vi "Logging Tree Contains.vi"(2 "Name":string, 3 "TreeRef":refnum<vi>) -> (0 "Contained":bool, 1 "TreeRef":refnum<vi>)   [LabVIEW 2012]
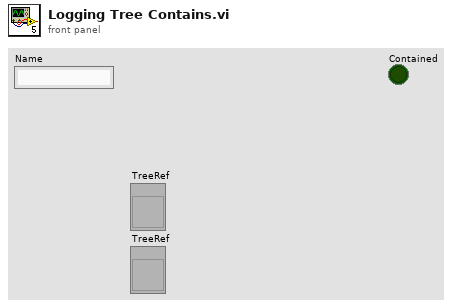
[diagram p1: front panel]
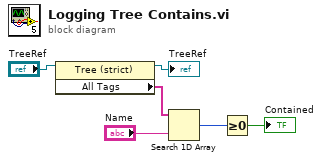
[diagram p0: block diagram]
diagram:
  n1 = property class="Tree (strict)"(reference="TreeRef") -> (reference out=→"TreeRef":refnum<vi>, "All Tags"=w4:string[])  [unwired: 1 in, 1 out]
  n2 = Search 1D Array(1D array=w4, element="Name") -> (index of element=w2:i32)  [unwired: 1 in]
  n3 = Greater Or Equal To 0?(x=w2) -> (x >= 0?=→"Contained":bool)
